vi "Write Measurement Name.vi"(10 "Measurement Name":string, 11 "Find Devices of Specified Type Msg in":refnum<class "Find Devices of Specified Type Msg.lvclass">) -> (3 "Find Devices of Specified Type Msg out":refnum<class "Find Devices of Specified Type Msg.lvclass">)   [LabVIEW 2016, in "Controller Actor.lvlib" / "Find Devices of Specified Type Msg.lvclass"]
uses:
  Find Devices of Specified Type Msg.lvclass
  Find Devices of Specified Type Msg.lvclass/Find Devices of Specified Type Msg.ctl
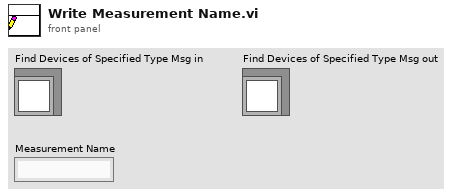
[diagram p1: front panel]
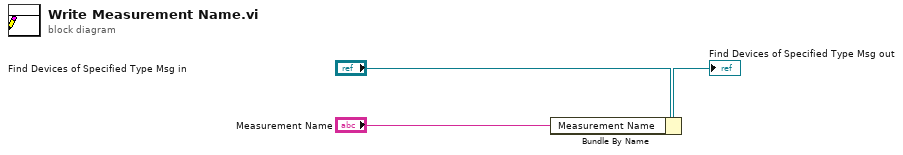
[diagram p0: block diagram]
diagram:
  n1 = Bundle By Name(cluster="Find Devices of Specified Type Msg in", "Measurement Name"="Measurement Name") -> (→"Find Devices of Specified Type Msg out":refnum<class "Find Devices of Specified Type Msg.lvclass">)
